vi "Challenge_POSE_3D_STL_Picture.vi"() -> ()   [LabVIEW 2013]
doc: "This VI demonstrates how the order in which you apply transformations to an object in a 3D scene affects the object's position and orientation within the scene. \n\n<b>Rotate then Translate:</b>\nIf you apply a rotation to an object as the first transformation, the object rotates around its parent's axis, which exists in spatially the same place as the object's own axis. Regardless of what transformations follow the rotation, the object appears to rotate around its own axis. If you apply a translation after the rotation, the object appears offset from its parent and still spinning around its own axis.\n\n<b>Translate then Rotate:</b>\nIf you apply a translation to an object as the first transformation, the object still appears offset from its parent. However, if you then apply a rotation to the object, the object rotates around its parent by the angle you specify with the Translate Object VI."
panel:
  in  "POSE":dbl[](array[knob])=[0.0, 0.0, 0.0, 0.0, 0.0, 0.0] scale=0.0..90.0
  in  "Stop":bool
  out "3D Picture":refnum<vi>(3d-picture)
  # "Position and Orientation POSE"
  # "X"
  # "Y"
  # "Z"
  # "Rot X"
  # "Rot Y"
  # "XYZ --> Mobile frame\nZYX --> Fixed frame"
  # "Rot Z"
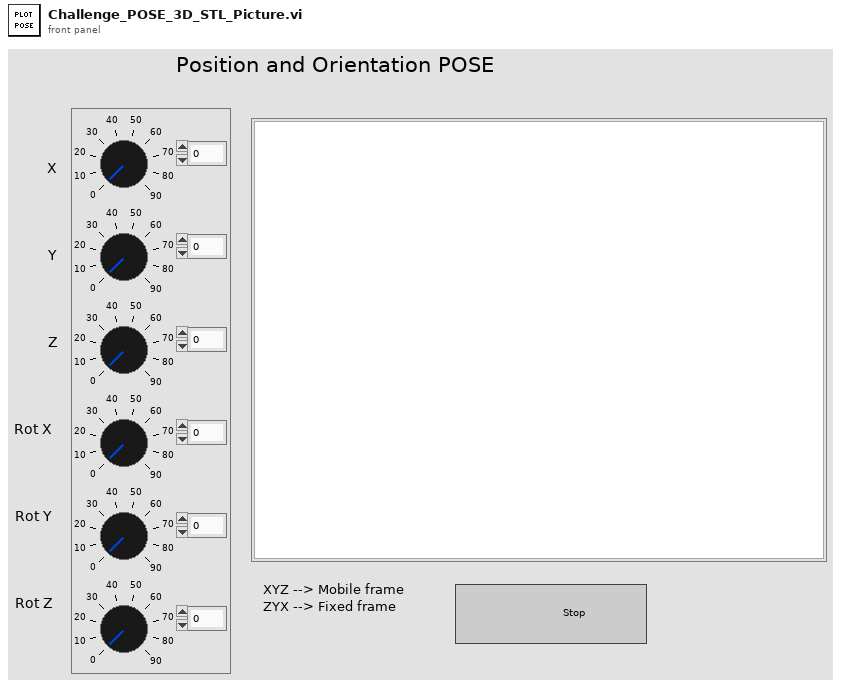
[diagram p1: front panel]
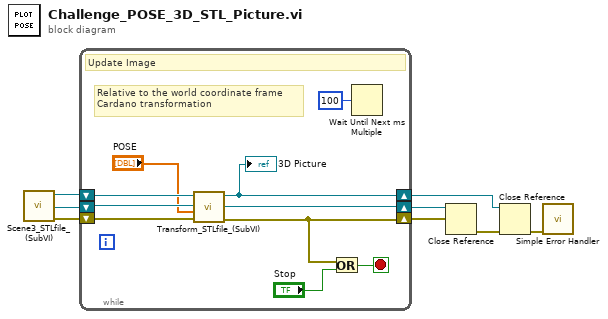
[diagram p0: block diagram]
diagram:
  n1 = call "Scene3_STLfile_(SubVI).vi"() -> ("error out"=w1:errorcluster, "New Object Out"=w2:refnum<vi>, "SceneObject out"=w3:refnum<vi>)  [unwired: 9 in]
  n2 = while {
    shift-right: [w9] -> w7
    shift-left: w1 -> [w12]
    shift-right: [w10] -> w4
    shift-left: w2 -> [w14]
    shift-right: [w11] -> w8
    shift-left: w3 -> [w15]
    stop <- w17 stop-if-true
    # "Relative to the world coordinate frame \nCardano transformation"
    # "Update Image"
    n3 = call "Transform_STLfile_(SubVI).vi"("error in (no error)"=w12, "POSE"="POSE", "New Object In"=w14, "SceneObject In"=w15) -> ("error out"=w9:errorcluster, "New Object out"=w10:refnum<vi>, "SceneObject Out"=w11:refnum<vi>)  [unwired: 5 in]
    "3D Picture" <- w11
    n4 = Or(x=w9, y="Stop") -> (x .or. y?=w17:bool)
    n5 = Wait Until Next ms Multiple(millisecond multiple=u32 100 ("milliseconds to wait")) -> ()  [unwired: 1 out]
  }
  n6 = Close Reference(reference=w4, error in (no error)=w7) -> (error out=w5:errorcluster)
  n7 = Close Reference(reference=w8, error in (no error)=w5) -> (error out=w6:errorcluster)
  n8 = call <vilib>:"Simple Error Handler.vi"("error in (no error)"=w6) -> ()  [unwired: 4 in, 5 out]
